vi "LuaVIEW Prepare Task.vi"(0 "script file or name (no name)":path, 5 "custom search directory (none)":path, 7 "script string (\"\" == load from file)":string, 9 "launch mode (whatever)":enum16{"asynchronous", "manual", "synchronous"}(ring), 11 "error in (no error)":errorcluster, 12 "identifier (none)":string, 13 "swap? (false)":bool) -> (4 "identifier":string, 8 "task instance":refnum<vi>, 15 "error out":errorcluster)   [LabVIEW 2012]
doc: "Prepare a new LuaVIEW task. Loads and preprocesses the task script and any import scripts, opens a LuaVIEW state, compiles the script(s), instantiates the task VI if necessary, and makes the preparations (task info and scripts info(s)) available to the task context."
uses:
  typedefs/clusters/LuaVIEW Script Info.ctl
  typedefs/t_LuaVIEW Prepared Script Infos Methods.ctl
  typedefs/t_LuaVIEW Task Signals.ctl
  typedefs/t_LuaVIEW Task Modes.ctl
  typedefs/t_LuaVIEW CIN Spinlocked Actions.ctl
  typedefs/t_LuaVIEW Task List Methods.ctl
  glb_LuaVIEW Configuration Globals.vi
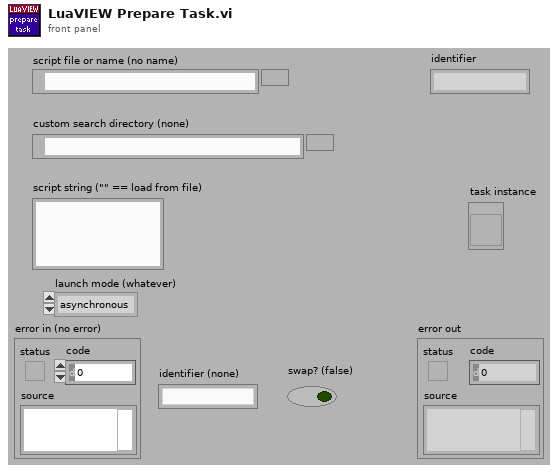
[diagram p1: front panel]
types:
  T1 = typedef "LuaVIEW Script Info.ctl" = cluster{"path":path, "description":string, "text":string, "parent index":i32, "version":string}
  T2 = typedef "t_LuaVIEW Prepared Script Infos Methods.ctl" = enum16{"isempty?", "empty", "set", "discard"}
  T3 = typedef "t_LuaVIEW Task List Methods.ctl" = enum16{"clear list", "add", "test", "remove", "get ref", "get task info", "get list", "get script info", "ongoing?", "resume", "pause", "stop", "confirm", "message"}
  T4 = typedef "t_LuaVIEW CIN Spinlocked Actions.ctl" = enum16{"totals", "taskcount", "open", "registerpublic", "registerexport", "revokeexports", "unregnextpublic", "usepublic", "pollexport", "close", "startyieldtest", "endyieldtest", "pollprintbuffer"}
  T5 = typedef "t_LuaVIEW Task Signals.ctl" = enum32{"resume", "pause", "swap", "stop", "confirm"}
  T6 = typedef "t_LuaVIEW Task Modes.ctl" = enum16{"initializing", "running", "executing", "paused", "error", "swapping"}
  T7 = typedef "LuaVIEW Task Info.ctl" = cluster{"main script":string, "identifier":string, "class":string, "description":string, "mode":T6, "handler":string, "LuaVIEW reference":T8, "scripts":i32, "hide":bool, "active":bool, "error msg":string, "defer":bool, "launch":enum16{"asynchronous", "manual", "synchronous"}, "main path valid":bool, "start time":dbl, "swap time":dbl, "task VI":refnum<vi>, "prefsys":enum32{"invalid execution system", "user interface", "standard", "instrument i/o", "data acquisition", "other 1", "other 2", "same as caller"}, "priority":enum32{"invalid priority", "background priority", "normal priority", "above normal priority", "high priority", "time critical priority", "subroutine"}, "signal flags":u32, "allow mask":u32, "handle mask":u32, "disallow manual":bool}
  T8 = typedef "t_LuaVIEW Reference.ctl" = refnum<k1>
  T9 = enum32{"invalid priority", "background priority", "normal priority", "above normal priority", "high priority", "time critical priority", "subroutine"}
  T10 = enum32{"invalid execution system", "user interface", "standard", "instrument i/o", "data acquisition", "other 1", "other 2", "same as caller"}
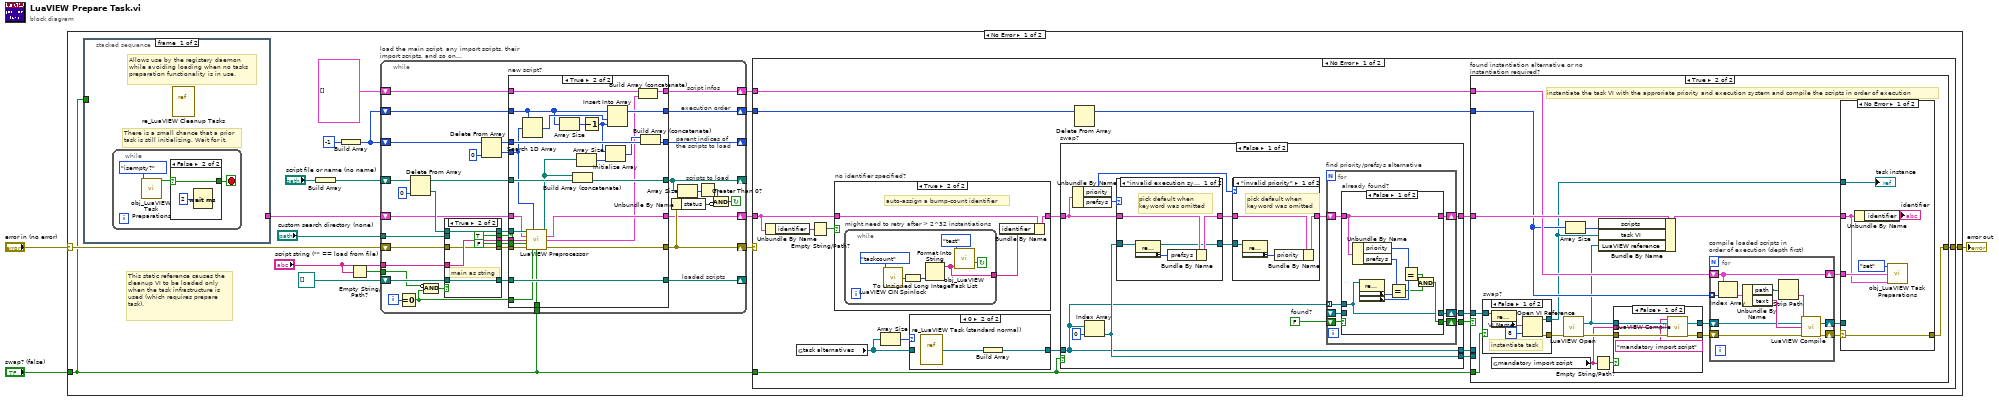
[diagram p0: block diagram]
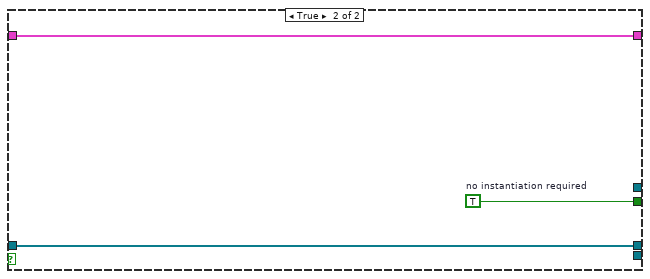
[diagram p5: hidden frame]
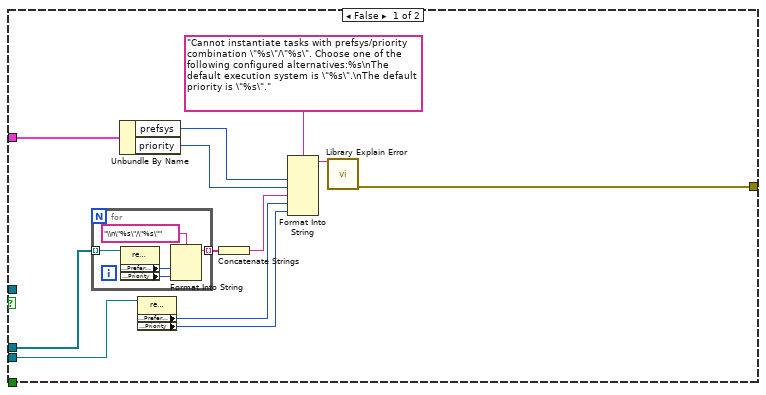
[diagram p6: hidden frame]
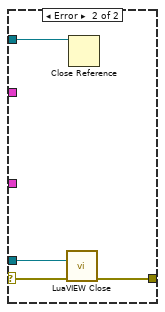
[diagram p9: hidden frame]
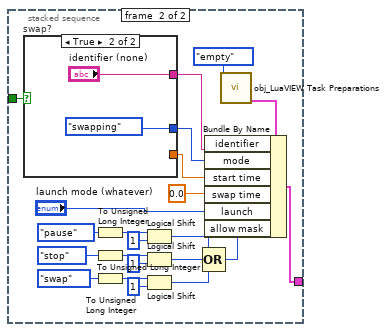
[diagram p14: hidden frame]
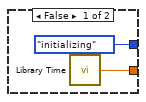
[diagram p15: hidden frame]
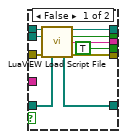
[diagram p16: hidden frame]
diagram:
  n1 = case shown="No Error" "error in (no error)" {
    selector: "error in (no error)" -> [w11 w286]
    tunnel: [w6 w286] -> w3
    tunnel: "swap? (false)" -> [w5 _]
    frame No Error {
      # "This static reference causes the\ncleanup VI to be loaded only\nwhen the task infrastructure is\nused (which requires prepare\ntask)."
      n2 = stacked-sequence {
        tunnel: [_ w193] -> w12
        tunnel: w5 -> [_ w192]
        frame #0 {
          # "Allows use by the registery daemon\nwhile avoiding loading when no tasks\npreparation functionality is in use."
          # "There is a small chance that a prior\ntask is still initializing. Wait for it."
          n3 = while {
            stop <- w169 stop-if-true
            n4 = call "obj_LuaVIEW Task Preparations.vi"("method"=t_LuaVIEW_Prepared_Script_Infos_Methods."isempty?") -> ("empty?"=w168:bool)  [unwired: 12 in, 2 out]
            n5 = case shown="False" w168 {
              tunnel: [w171 w173] -> w169
              selector: w168 -> [w171 w173]
              frame True {
              }
              frame False {
                n6 = Wait (ms)(milliseconds to wait=u32 2) -> ()  [unwired: 1 out]
              }
            }
          }
          n7 = vi-ref "re_LuaVIEW Cleanup Tasks.vi"() -> ()  [unwired: 1 out]
        }
        frame #1 {
          n8 = case "swap?" shown="True" w192 {
            tunnel: [_ "identifier (none)"] -> w175
            tunnel: [w197 _] -> w182
            tunnel: [t_LuaVIEW_Task_Modes."initializing" ("mode") t_LuaVIEW_Task_Modes."swapping" ("mode")] -> w174
            frame False {
              n9 = call "Library Time.vi"() -> ("time"=w197:dbl)  [unwired: 1 in]
            }
            frame True {
            }
          }
          n10 = To Unsigned Long Integer(number=t_LuaVIEW_Task_Signals."pause" ("signal")) -> (unsigned 32bit integer=w185:u32)
          n11 = To Unsigned Long Integer(number=t_LuaVIEW_Task_Signals."stop" ("signal")) -> (unsigned 32bit integer=w189:u32)
          n12 = To Unsigned Long Integer(number=t_LuaVIEW_Task_Signals."swap" ("signal")) -> (unsigned 32bit integer=w178:u32)
          n13 = Logical Shift(y=w185, x=u32 1) -> (x << y=w186:u32)
          n14 = Logical Shift(y=w189, x=u32 1) -> (x << y=w191:u32)
          n15 = Logical Shift(y=w178, x=u32 1) -> (x << y=w176:u32)
          n16 = Compound Arithmetic op=OR(w186, w191, w176) -> (w183:u32)
          n17 = call "obj_LuaVIEW Task Preparations.vi"("method"=t_LuaVIEW_Prepared_Script_Infos_Methods."empty") -> ("task info out"=w194:T7)  [unwired: 12 in, 2 out]
          n18 = Bundle By Name(cluster=w194, "identifier"=w175, "mode"=w174, "start time"=w182, "swap time"=0.0, "launch"="launch mode (whatever)", "allow mask"=w183) -> (w193:T7)
        }
      }
      n19 = Build Array("script file or name (no name)") -> (w19:path[])
      n20 = Build Array(-1) -> (w17:i32[])
      n21 = Empty String/Path?(string/path="script string (\"\" == load from file)") -> (empty?=w16:bool)
      n22 = while "load the main script, any import scripts, their import scripts, and so on..." {
        shift-right: [w232] -> w4
        shift-left: w11 -> [w215]
        shift-right: [w229] -> _
        shift-left: path[] [] ("loaded scripts out") -> [w230]
        shift-right: [w222] -> _
        shift-left: w19 -> [w226]
        shift-right: [w227] -> _
        shift-left: w17 -> [w224]
        shift-right: [w216] -> w8
        shift-left: w17 -> [w217]
        tunnel: "custom search directory (none)" -> [w213]
        tunnel: "script string (\"\" == load from file)" -> [w210]
        tunnel: w16 -> [w211]
        shift-right: [w203] -> w10
        shift-left: w12 -> [w204]
        shift-right: [w201] -> w7
        shift-left: T1[] [] -> [w202]
        tunnel: w5 -> [w200]
        i -> [w214]
        stop <- w235 continue-if-true
        # "script infos"
        # "execution order"
        # "loaded scripts"
        # "scripts to load"
        # "parent indices of\nthe scripts to load"
        n23 = Equal To 0?(x=w214) -> (x = 0?=w209:bool)
        n24 = Delete From Array(array=w226, index=0) -> (deleted portion=w221:path, array with subset deleted=w225:path[])  [unwired: 1 in]
        n25 = Compound Arithmetic op=AND(invert w211, w209) -> (w212:bool)
        n26 = case shown="True" w212 {
          tunnel: [w246 TRUE ("have new script")] -> w231
          tunnel: w230 -> [w245 w251]
          tunnel: [w244 w251] -> w228
          tunnel: w221 -> [w243 w249]
          tunnel: w215 -> [w242 w248]
          tunnel: [w241 w248] -> w207
          tunnel: [w240 w252] -> w206
          tunnel: [w239 w249] -> w205
          tunnel: w213 -> [w238 _]
          tunnel: w210 -> [_ w252]
          tunnel: [TRUE ("have new script") FALSE ("have new script")] -> w208
          frame False {
            n27 = call "LuaVIEW Load Script File.vi"("script file"=w243, "custom search directory (none)"=w238, "error in (no error)"=w242, "loaded scripts in (none)"=w245) -> ("absolute path"=w239:path, "have new script"=w246:bool, "script text"=w240:string, "loaded scripts out"=w244:path[], "error out"=w241:errorcluster)  [unwired: 7 in]
          }
          frame True {
            # "main as string"
          }
        }
        n28 = Delete From Array(array=w224, index=0) -> (deleted portion=w220:i32, array with subset deleted=w223:i32[])  [unwired: 1 in]
        n29 = case "new script?" shown="True" w231 {
          tunnel: w206 -> [_ w285]
          tunnel: w207 -> [w258 w284]
          tunnel: [w258 w270] -> w232
          tunnel: [w259 w274] -> w229
          tunnel: w228 -> [w259 w274]
          tunnel: w225 -> [w256 w283]
          tunnel: [w256 w282] -> w222
          tunnel: w223 -> [w257 w281]
          tunnel: [w257 w278] -> w227
          tunnel: w220 -> [_ w264]
          tunnel: w217 -> [w255 w271]
          tunnel: [w255 w275] -> w216
          tunnel: w209 -> [_ w269]
          tunnel: w208 -> [_ w268]
          tunnel: w205 -> [_ w267]
          tunnel: w204 -> [w254 w265]
          tunnel: [w254 w266] -> w203
          tunnel: w202 -> [w253 w263]
          tunnel: [w253 w262] -> w201
          tunnel: w200 -> [_ w260]
          frame False {
          }
          frame True {
            n30 = Search 1D Array(1D array=w271, element=w264) -> (index of element=w276:i32)  [unwired: 1 in]
            n31 = call "LuaVIEW Preprocessor.vi"("path"=w267, "parent index"=w264, "task info in"=w265, "script"=w285, "main path valid?"=w268, "error in (no error)"=w284, "main script?"=w269, "swap? (false)"=w260) -> ("import paths"=w279:path[], "task info out"=w266:T7, "script info"=w261:T1, "error out"=w270:errorcluster)  [unwired: 4 in]
            n32 = Array Size(array=w271) -> (size(s)=w272:i32)
            n33 = Build Array (concatenate)(w279, w283) -> (w282:path[])
            n34 = Array Size(array=w279) -> (size(s)=w280:i32)
            n35 = Decrement(x=w272) -> (x-1=w273:i32)
            n36 = Initialize Array(w273, w280) -> (w277:i32[])
            n37 = Insert Into Array(array=w271, index=w276, new element=w273) -> (w275:i32[])
            n38 = Build Array (concatenate)(w263, w261) -> (w262:T1[])
            n39 = Build Array (concatenate)(w277, w281) -> (w278:i32[])
          }
        }
        n40 = Unbundle By Name(w232) -> ("status"=w234:bool)
        n41 = Array Size(array=w222) -> (size(s)=w236:i32)
        n42 = Greater Than 0?(x=w236) -> (x > 0?=w233:bool)
        n43 = Compound Arithmetic op=AND(w233, invert w234) -> (w235:bool)
      }
      n44 = case shown="No Error" w4 {
        selector: w4 -> [_ w167]
        tunnel: w10 -> [w29 _]
        tunnel: w8 -> [w37 _]
        tunnel: w7 -> [w36 _]
        tunnel: [w35 w167] -> w6
        tunnel: w5 -> [w34 _]
        frame No Error {
          n45 = Unbundle By Name(w29) -> ("identifier"=w28:string)
          n46 = global read "glb_LuaVIEW Configuration Globals.vi" "task alternatives"() -> (w33:refnum<vi>[])
          n47 = Empty String/Path?(string/path=w28) -> (empty?=w30:bool)
          n48 = case "no identifier specified?" shown="True" w30 {
            tunnel: w29 -> [w154 w157]
            tunnel: [w154 w156] -> w27
            frame False {
            }
            frame True {
              # "auto-assign a bump-count identifier"
              n49 = while "might need to retry after > 2^32 instantiations" {
                tunnel: [w158] -> w155
                stop <- w159 continue-if-true
                n50 = call "LuaVIEW CIN Spinlock.vi"("action"=t_LuaVIEW_CIN_Spinlocked_Actions."taskcount") -> ("index out"=w162:i32)  [unwired: 8 in, 6 out]
                n51 = To Unsigned Long Integer(number=w162) -> (unsigned 32bit integer=w163:u32)
                n52 = Format Into String(w163) -> (resulting string=w158:string)  [unwired: 3 in, 1 out]
                n53 = call "obj_LuaVIEW Task List.vi"("method"=t_LuaVIEW_Task_List_Methods."test", "task identifier"=w158) -> ("set/ongoing"=w159:bool)  [unwired: 8 in, 5 out]
              }
              n54 = Bundle By Name(cluster=w157, "identifier"=w155) -> (w156:T7)
            }
          }
          n55 = Array Size(array=w33) -> (size(s)=w32:i32)
          n56 = case shown="0" w32 {
            tunnel: [w164 w165] -> w31
            tunnel: w33 -> [w164 _]
            frame Default {
            }
            frame 0 {
              n57 = vi-ref "re_LuaVIEW Task (standard normal).vi"() -> ("vi reference"=w166:refnum<vi>)
              n58 = Build Array(w166) -> (w165:refnum<vi>[])
            }
          }
          n59 = case "swap?" shown="False" w34 {
            tunnel: w27 -> [w48 w82]
            tunnel: [w42 w83] -> w26
            tunnel: [w41 w82] -> w25
            tunnel: w31 -> [w38 w84]
            tunnel: [w40 _] -> w24
            tunnel: [w39 _] -> w23
            tunnel: [w38 w84] -> w21
            frame False {
              w43 = FALSE  # found?
              n60 = Unbundle By Name(w48) -> ("priority"=w46:T9, "prefsys"=w49:T10)
              n61 = Index Array(array=w38, index=0) -> (element=w39:refnum<vi>)
              n62 = case shown="\"invalid execution system\"" w49 {
                tunnel: w39 -> [w79 w80]
                tunnel: w48 -> [w78 w81]
                tunnel: [w76 w81] -> w47
                tunnel: [w75 w80] -> w45
                frame "invalid execution system" {
                  # "pick default when\nkeyword was omitted"
                  n63 = property class="re_LuaVIEW Task (normal standar"(reference=w79) -> (reference out=w75:refnum<vi>, "Execution:Preferred Exec System"=w77:T10)  [unwired: 1 in, 1 out]
                  n64 = Bundle By Name(cluster=w78, "prefsys"=w77) -> (w76:T7)
                }
                frame Default {
                }
              }
              n65 = case shown="\"invalid priority\"" w46 {
                tunnel: w45 -> [w73 _]
                tunnel: w47 -> [w72 w74]
                tunnel: [w70 w74] -> w44
                frame "invalid priority" {
                  # "pick default when\nkeyword was omitted"
                  n66 = property class="re_LuaVIEW Task (normal standar"(reference=w73) -> ("Execution:Priority"=w71:T9)  [unwired: 1 in, 2 out]
                  n67 = Bundle By Name(cluster=w72, "priority"=w71) -> (w70:T7)
                }
                frame Default {
                }
              }
              n68 = for "find priority/prefsys alternative" {
                shift-right: [w53] -> w41
                shift-left: w44 -> [w57]
                tunnel: w38 -> [w56] mode=indexing
                shift-right: [w54] -> w42
                shift-left: w43 -> [w55]
                shift-right: [w52] -> w40
                shift-left: _ -> [w51]
                n69 = case "already found?" shown="False" w55 {
                  selector: w55 -> [_ w69]
                  tunnel: w57 -> [w60 w68]
                  tunnel: w56 -> [w58 _]
                  tunnel: [w59 w69] -> w54
                  tunnel: [w60 w68] -> w53
                  tunnel: [w58 w67] -> w52
                  tunnel: w51 -> [_ w67]
                  frame False {
                    n70 = Unbundle By Name(w60) -> ("priority"=w66:T9, "prefsys"=w63:T10)
                    n71 = property class="re_LuaVIEW Task (normal standar"(reference=w58) -> ("Execution:Preferred Exec System"=w64:T10, "Execution:Priority"=w65:T9)  [unwired: 1 in, 2 out]
                    n72 = Equal?(x=w63, y=w64) -> (x = y?=w61:bool)
                    n73 = Equal?(x=w66, y=w65) -> (x = y?=w62:bool)
                    n74 = And(x=w62, y=w61) -> (x .and. y?=w59:bool)
                  }
                  frame True {
                  }
                }
              }
            }
            frame True {
              w83 = TRUE  # no instantiation required
            }
          }
          n75 = Delete From Array(array=w37) -> (array with subset deleted=w22:i32[])  [unwired: 2 in, 1 out]
          n76 = case "found instantiation alternative or no instantiation required?" shown="True" w26 {
            tunnel: w25 -> [w94 w119]
            tunnel: w21 -> [w91 _]
            tunnel: w24 -> [_ w120]
            tunnel: [w90 w117] -> w35
            tunnel: w23 -> [w87 _]
            tunnel: w36 -> [_ w114]
            tunnel: w22 -> [_ w112]
            tunnel: w34 -> [_ w104]
            frame False {
              n77 = for {
                tunnel: w91 -> [w101] mode=indexing
                tunnel: [w97] -> w89 mode=indexing
                n78 = property class="re_LuaVIEW Task (normal standar"(reference=w101) -> ("Execution:Preferred Exec System"=w100:T10, "Execution:Priority"=w98:T9)  [unwired: 1 in, 2 out]
                n79 = Format Into String(format string="\\n\"%s\"/\"%s\"", w100, w98) -> (resulting string=w97:string)  [unwired: 2 in, 1 out]
              }
              n80 = Unbundle By Name(w94) -> ("prefsys"=w93:T10, "priority"=w92:T9)
              n81 = property class="re_LuaVIEW Task (normal standar"(reference=w87) -> ("Execution:Preferred Exec System"=w86:T10, "Execution:Priority"=w85:T9)  [unwired: 1 in, 2 out]
              n82 = Concatenate Strings(w89) -> (w88:string)
              n83 = Format Into String(format string="Cannot instantiate tasks with prefsys/priority combination \"%s\"/\"%s\". Choose one of the following configured alternatives:%s\nThe default execution system is \"%s\".\nThe default priority is \"%s\".", w93, w92, w88, w86, w85) -> (resulting string=w95:string)  [unwired: 2 in, 1 out]
              n84 = call "Library Explain Error.vi"("explanation prefix (none)"=w95) -> ("explained error"=w90:errorcluster)  [unwired: 14 in]
            }
            frame True {
              # "instantiate the task VI with the approriate priority and execution system and compile the scripts in order of execution"
              n85 = case "swap?" shown="False" w104 {
                tunnel: w120 -> [w123 _]
                tunnel: [w122 _] -> w118
                tunnel: [w121 _] -> w103
                frame False {
                  # "instantiate task"
                  n86 = property class="re_LuaVIEW Task (normal standar"(reference=w123) -> ("VI Name"=w124:string)  [unwired: 1 in, 2 out]
                  n87 = Open VI Reference(vi path=w124, options=8) -> (vi reference=w121:refnum<vi>, error out=w122:errorcluster)  [unwired: 4 in]
                }
                frame True {
                }
              }
              n88 = global read "glb_LuaVIEW Configuration Globals.vi" "mandatory import script"() -> (w107:string)
              n89 = call "LuaVIEW Open.vi"("error in (no error)"=w118) -> ("LuaVIEW reference"=w102:T8, "error out"=w108:errorcluster)  [unwired: 13 in]
              n90 = Array Size(array=w112) -> (size(s)=w116:i32)
              n91 = Empty String/Path?(string/path=w107) -> (empty?=w109:bool)
              n92 = Bundle By Name(cluster=w119, "scripts"=w116, "task VI"=w103, "LuaVIEW reference"=w102) -> (w115:T7)
              n93 = case shown="False" w109 {
                tunnel: w107 -> [w131 _]
                tunnel: w108 -> [w130 w133]
                tunnel: w102 -> [w129 w132]
                tunnel: [w127 w132] -> w106
                tunnel: [w126 w133] -> w105
                frame False {
                  n94 = call "LuaVIEW Compile.vi"("script name"="mandatory import script", "LuaVIEW reference in"=w129, "script"=w131, "error in (no error)"=w130) -> ("LuaVIEW reference out"=w127:T8, "error out"=w126:errorcluster)  [unwired: 10 in]
                }
                frame True {
                }
              }
              n95 = for "compile loaded scripts in\norder of execution (depth first)" {
                shift-right: [w139] -> w113
                shift-left: w105 -> [w140]
                shift-right: [w134] -> w110
                shift-left: w114 -> [w134]
                tunnel: w112 -> [w138] mode=indexing
                shift-right: [w136] -> w111
                shift-left: w106 -> [w137]
                n96 = Index Array(array=w134, index=w138) -> (element=w135:T1)
                n97 = Unbundle By Name(w135) -> ("path"=w142:path, "text"=w141:string)
                n98 = Strip Path(path=w142) -> (name=w143:string)  [unwired: 1 out]
                n99 = call "LuaVIEW Compile.vi"("script name"=w143, "LuaVIEW reference in"=w137, "script"=w141, "error in (no error)"=w140) -> ("LuaVIEW reference out"=w136:T8, "error out"=w139:errorcluster)  [unwired: 10 in]
              }
              n100 = case shown="No Error" w113 {
                selector: w113 -> [w149 w151]
                tunnel: w103 -> [w144 w153]
                tunnel: [w149 w150] -> w117
                tunnel: w115 -> [w145 _]
                tunnel: w111 -> [_ w152]
                tunnel: w110 -> [w146 _]
                frame No Error {
                  n101 = Unbundle By Name(w145) -> ("identifier"=→"identifier":string)
                  n102 = call "obj_LuaVIEW Task Preparations.vi"("method"=t_LuaVIEW_Prepared_Script_Infos_Methods."set", "script infos in"=w146, "task info in"=w145) -> ()  [unwired: 10 in, 3 out]
                  "task instance" <- w144
                }
                frame Error {
                  n103 = call "LuaVIEW Close.vi"("LuaVIEW reference"=w152, "error in (no error)"=w151) -> ("dup error"=w150:errorcluster)  [unwired: 13 in]
                  n104 = Close Reference(reference=w153) -> ()  [unwired: 1 in, 1 out]
                }
              }
            }
          }
        }
        frame Error {
        }
      }
    }
    frame Error {
    }
  }
  "error out" <- w3
